vi "Simulador Circuito RLC- Gullit e Gabriela.vi"() -> ()   [LabVIEW 2020]
uses:
  <vilib>/Utility/file.llb/Read Delimited Spreadsheet (DBL).vi
  <vilib>/measure/NI_MABase.lvlib
panel:
  in  "i'(0)":dbl=1.0
  in  "i(0)":dbl
  in  "Vc'(0)":dbl=1.0
  in  "Vc(0)":dbl
  in  "C":dbl
  in  "L":dbl
  in  "R":dbl
  in  "Gerar ondas\nde saída":bool
  out "Tensão no Capacitor":cluster{dbl[], "Y":dbl[]}[](graph)
  out "Corrente":cluster{dbl[], "Y":dbl[]}[](graph)
  in  "Arquivo texto da onda":path
  out "Onda de entrada":cluster{dbl[], "Y":dbl[]}(graph)
  in  "Duty Cicle":dbl
  in  "Informação da amostragem":T1={"Taxa de amostragem"=1000.0, "N° de amostras"=100000.0} {"N° de amostras" format="%#.6g"; "Taxa de amostragem" format="%#.6g"}
  in  "Gerar onda \nde Entrada":bool
  in  "Tipo de Onda":u16(ring) items=["Senoidal", "Quadrada", "Onda qualquer", ""]
  in  "Amplitude":dbl
  in  "Frequência":dbl
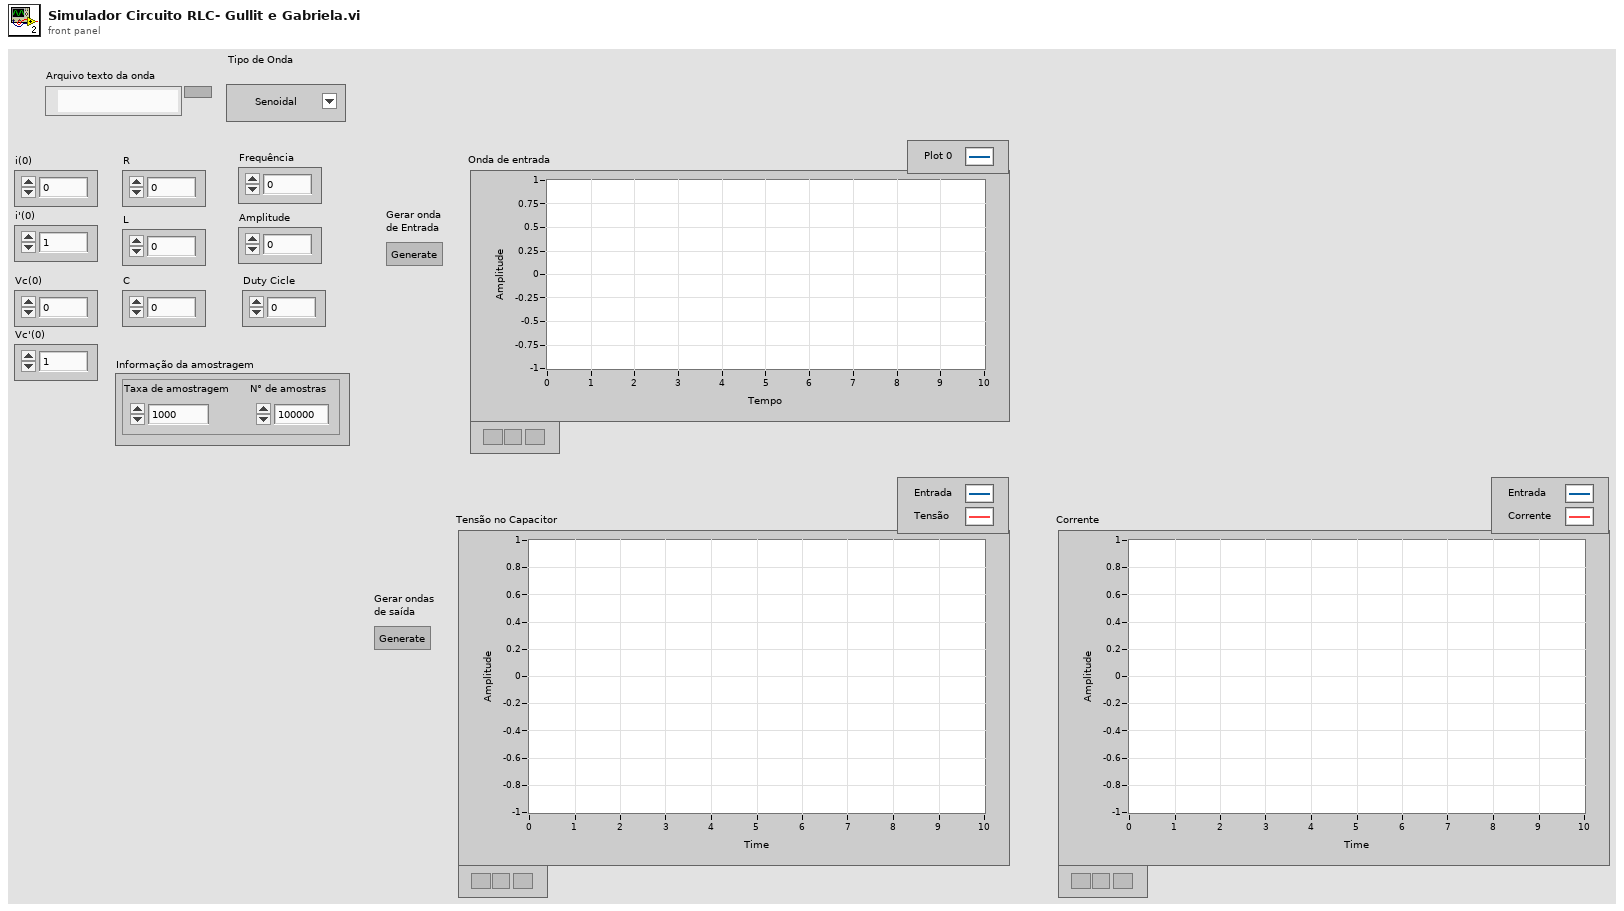
[diagram p1: front panel]
types:
  T1 = cluster{"Taxa de amostragem":dbl, "N° de amostras":dbl}
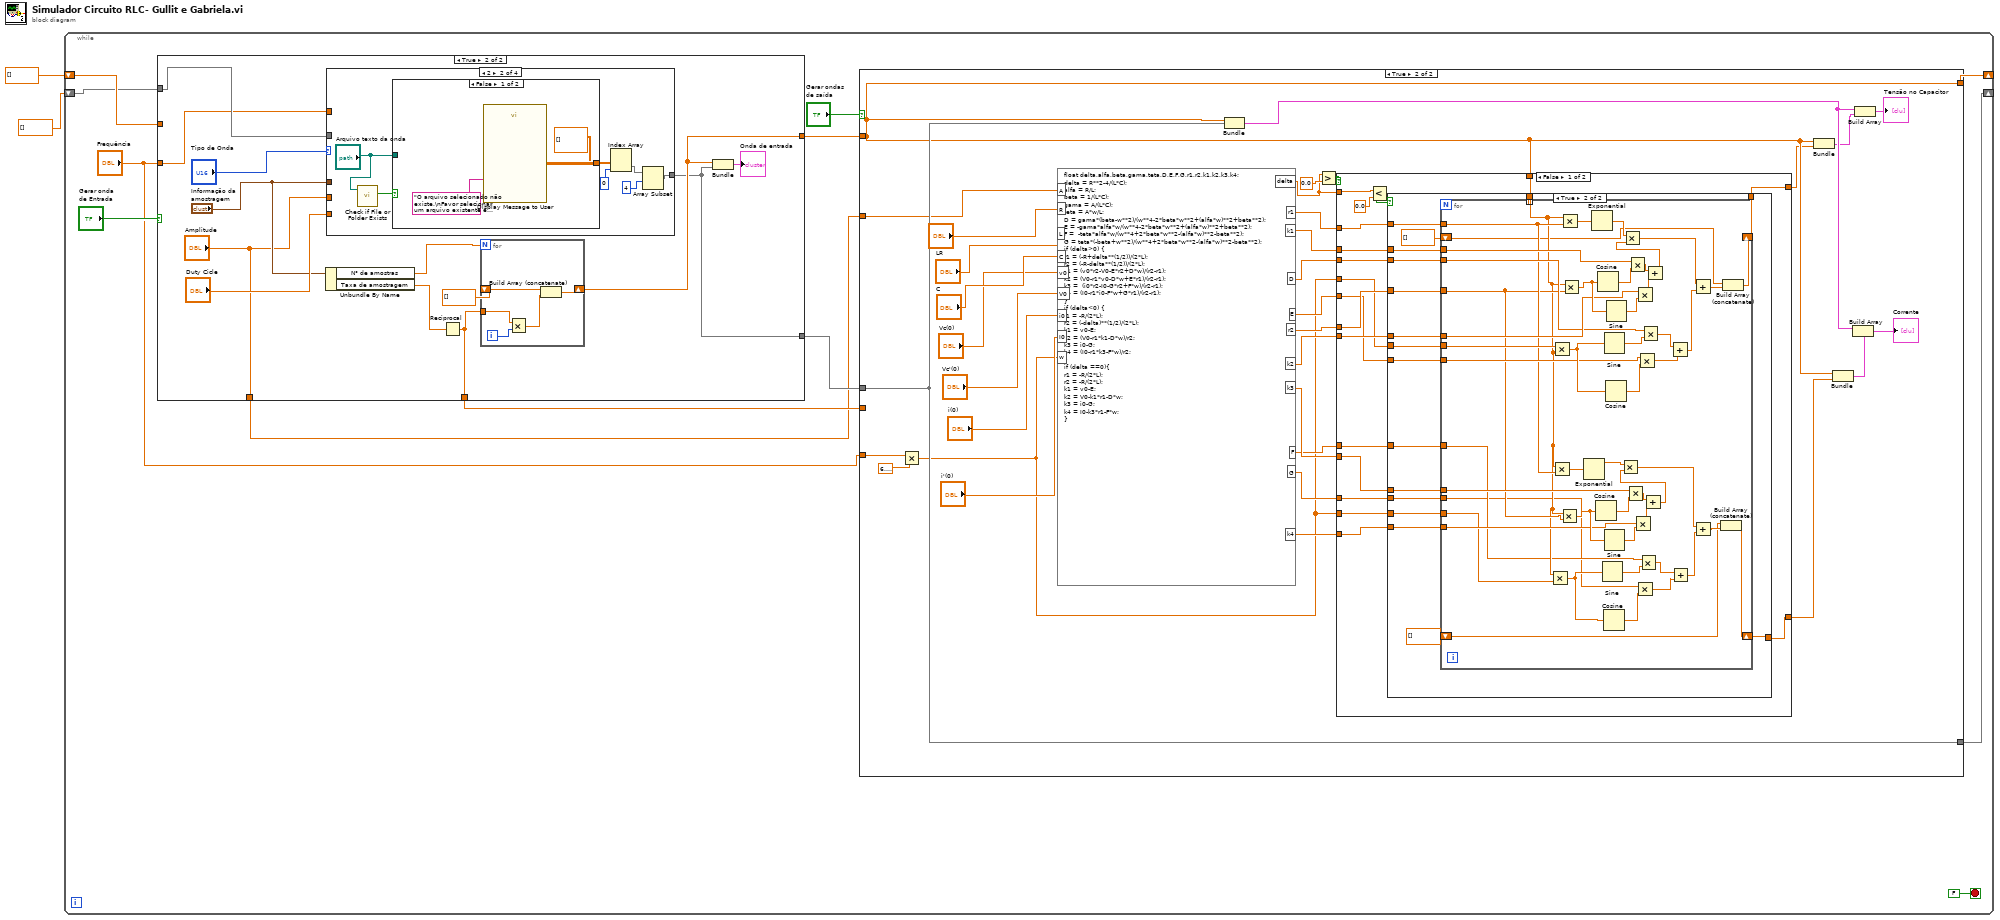
[diagram p0: block diagram]
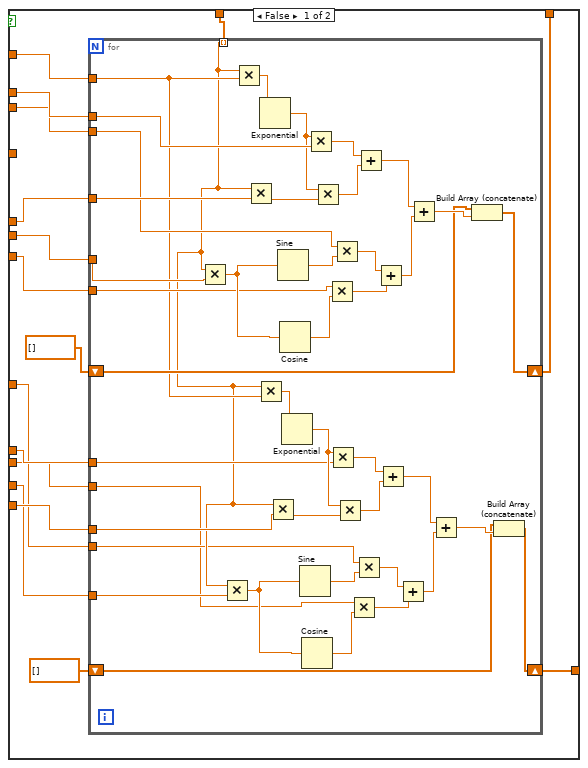
[diagram p3: hidden frame]
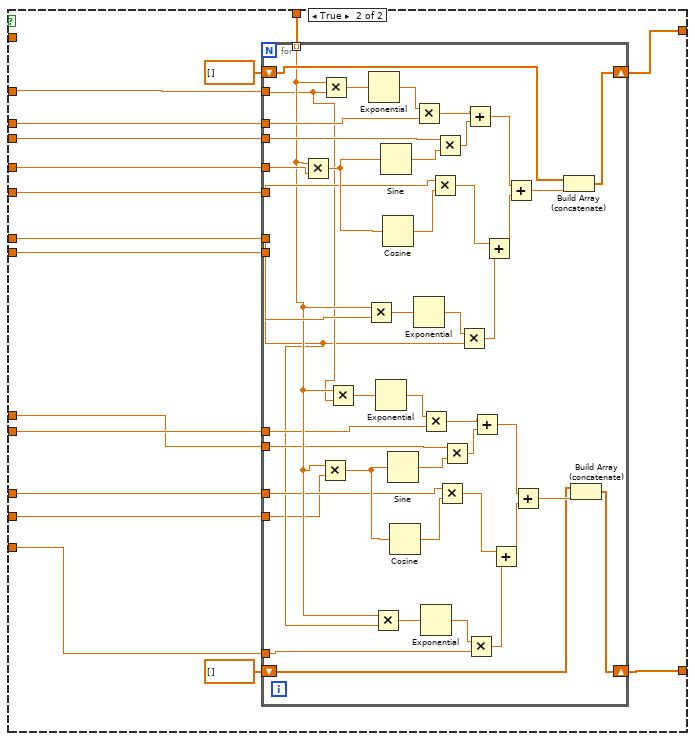
[diagram p4: hidden frame]
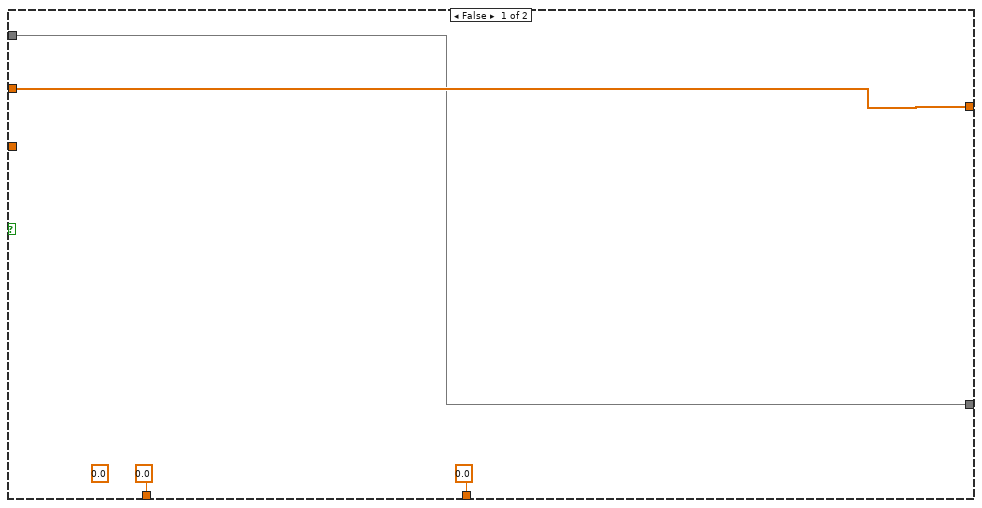
[diagram p5: hidden frame]
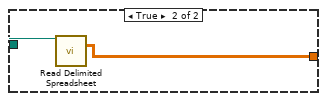
[diagram p7: hidden frame]
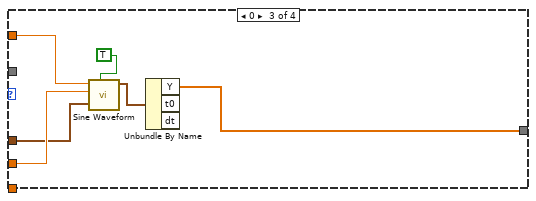
[diagram p8: hidden frame]
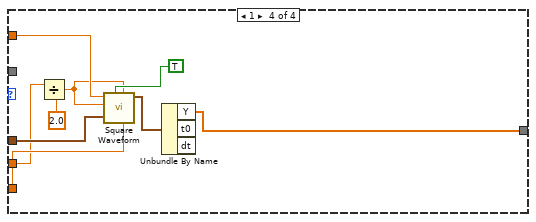
[diagram p9: hidden frame]
diagram:
  n1 = while {
    shift-right: [w10] -> _
    shift-left: dbl[] [] -> [w8]
    shift-right: [w9] -> _
    shift-left: dbl[] [] ("Y") -> [w7]
    stop <- FALSE stop-if-true
    n2 = case shown="True" "Gerar onda \nde Entrada" {
      tunnel: [w257 w264] -> w12
      tunnel: [w256 w263] -> w11
      tunnel: w8 -> [w257 _]
      tunnel: w7 -> [w256 w262]
      tunnel: [0.0 w260] -> w6
      tunnel: [0.0 ("Amplitude") "Amplitude"] -> w5
      tunnel: "Frequência" -> [_ w258]
      frame False {
        (unwired) 0.0 ("Frequência")
      }
      frame True {
        n3 = Unbundle By Name("Informação da amostragem") -> ("N° de amostras"=w266:dbl, "Taxa de amostragem"=w267:dbl)
        n4 = case shown="2" "Tipo de Onda" {
          tunnel: "Amplitude" -> [_ _ w292 w295]
          tunnel: w258 -> [_ _ w293 w302]
          tunnel: w262 -> [w276 _ _ _]
          tunnel: "Informação da amostragem" -> [_ _ w291 w301]
          tunnel: "Duty Cicle" -> [_ _ _ w300]
          tunnel: [w276 w279 w288 w297] -> w263
          frame Default {
          }
          frame 2 {
            n5 = call <vilib>:"Check if File or Folder Exists.vi"("path"="Arquivo texto da onda") -> ("file or folder exists?"=w277:bool)  [unwired: 8 in, 2 out]
            n6 = case shown="False" w277 {
              tunnel: "Arquivo texto da onda" -> [_ w287]
              tunnel: [dbl[][] [] ("all rows") w286] -> w281
              frame False {
                n7 = call "Display Message to User"("Message"="O arquivo selecionado não existe.\nFavor selecionar um arquivo existente e recomeçe a VI.") -> ()  [unwired: 9 in, 2 out]
              }
              frame True {
                n8 = call-poly <vilib>:"Read Delimited Spreadsheet.vi"("file path (dialog if empty)"=w287) -> ("all rows"=w286:dbl[][])  [unwired: 9 in, 5 out]
              }
            }
            n9 = Index Array(array=w281, index (col)=0 ("disabled index (col)")) -> (element=w282:dbl[])  [unwired: 1 in]
            n10 = Array Subset(array=w282, index=4) -> (w279:dbl[])  [unwired: 1 in]
          }
          frame 0 {
            n11 = call <vilib>:"Sine Waveform.vi"("sampling info"=w291, "reset signal"=TRUE, "amplitude"=w292, "frequency"=w293) -> ("signal out"=w289:waveform(dbl))  [unwired: 6 in, 1 out]
            n12 = Unbundle By Name(w289) -> ("Y"=w288:dbl[])  [unwired: 2 out]
          }
          frame 1 {
            n13 = Divide(x=w295, y=2.0) -> (x/y=w294:dbl)
            n14 = call <vilib>:"Square Waveform.vi"("duty cycle (%)"=w300, "offset"=w294, "sampling info"=w301, "reset signal"=TRUE, "amplitude"=w294, "frequency"=w302) -> ("signal out"=w298:waveform(dbl))  [unwired: 4 in, 1 out]
            n15 = Unbundle By Name(w298) -> ("Y"=w297:dbl[])  [unwired: 2 out]
          }
        }
        n16 = Reciprocal(x=w267) -> (1/x=w260:dbl)
        n17 = for {
          N: w266 -> [_]
          tunnel: w260 -> [w274]
          shift-right: [w272] -> w264
          shift-left: dbl[] [] -> [w271]
          i -> [w275]
          n18 = Multiply(x=w274, y=w275) -> (x*y=w273:dbl)
          n19 = Build Array (concatenate)(w271, w273) -> (w272:dbl[])
        }
        n20 = Bundle(w264, "Y"=w263) -> (→"Onda de entrada":cluster{dbl[], "Y":dbl[]})  [unwired: 1 in]
      }
    }
    n21 = case shown="True" "Gerar ondas\nde saída" {
      tunnel: w12 -> [w16 w37]
      tunnel: w11 -> [w15 w48]
      tunnel: [w16 w37] -> w10
      tunnel: [w15 w48] -> w9
      tunnel: w6 -> [_ _]
      tunnel: w5 -> [_ w42]
      tunnel: "Frequência" -> [_ w18]
      frame False {
      }
      frame True {
        n22 = Multiply(x=w18, y=6.283185307179586) -> (x*y=w17:dbl)
        n23 = formula code="float delta,alfa,beta,gama,teta,D,E,F,G,r1,r2,k1,k2,k3,k4;\ndelta = R**2-4/(L*C);\nalfa = R/L;\nbeta = 1/(L*C);\ngama = A/(L*C);\nteta = A*w/L;\nD = gama*(beta-w**2)/(w**4-2*beta*w**2+(alfa*w)**2+beta**2);\nE = -gama*alfa*w/(w**4-2*beta*w**2+(alfa*w)**2+beta**2);\nF =  -teta*alfa*w/(w**4+2*beta*w**2-(alfa*w)**2-beta**2);\nG = teta*(-beta+w**2)/(w**4+2*beta*w**2-(alfa*w)**2-beta**2);\nif (delta>0) {\nr1 = (-R+delta**(1/2))/(2*L);\nr2 = (-R-delta**(1/2))/(2*L);\nk1 = (v0*r2-V0-E*r2+D*w)/(r2-r1);\nk2 = (V0-r1*v0-D*w+E*r1)/(r2-r1);\nk3 =  (i0*r2-I0-G*r2+F*w)/(r2-r1);\nk4 = (I0-r1*i0-F*w+G*r1)/(r2-r1);\n}\nif (delta<0) {\nr1 = -R/(2*L);\nr2 = (-delta)**(1/2)/(2*L);\nk1 = v0-E;\nk2 = (V0-r1*k1-D*w)/r2;\nk3 = i0-G;\nk4 = (I0-r1*k3-F*w)/r2;\n}\nif (delta ==0){\nr1 = -R/(2*L);\nr2 = -R/(2*L);\nk1 = v0-E;\nk2 = V0-k1*r1-D*w;\nk3 = i0-G;\nk4 = I0-k3*r1-F*w;\n}"("C"="C", "L"="L", "R"="R", "A"=w42, "w"=w17, "v0"="Vc(0)", "V0"="Vc'(0)", "i0"="i(0)", "I0"="i'(0)") -> ("D"=w31:dbl, "E"=w32:dbl, "delta"=w24:dbl, "r1"=w36:dbl, "r2"=w34:dbl, "k1"=w35:dbl, "k2"=w33:dbl, "k3"=w28:dbl, "k4"=w25:dbl, "F"=w27:dbl, "G"=w26:dbl)
        n24 = Bundle(w37, "Y"=w48) -> (w49:cluster{dbl[], "Y":dbl[]})  [unwired: 1 in]
        n25 = Greater?(x=w24, y=0.0) -> (0:w40:bool)
        n26 = case shown="False" w40 {
          tunnel: w37 -> [w64 w208]
          tunnel: w36 -> [w63 w207]
          tunnel: w35 -> [w62 w206]
          tunnel: w34 -> [w61 w205]
          tunnel: w33 -> [w60 w204]
          tunnel: w17 -> [w59 w203]
          tunnel: w32 -> [w57 w202]
          tunnel: w31 -> [w58 w201]
          tunnel: w28 -> [w56 w199]
          tunnel: w27 -> [w53 w198]
          tunnel: w26 -> [w52 w197]
          tunnel: w25 -> [w54 w196]
          tunnel: w17 -> [w55 w194]
          tunnel: w24 -> [w66 _]
          tunnel: [w51 w193] -> w23
          tunnel: [w50 w192] -> w22
          frame False {
            n27 = Less?(x=w66, y=0.0) -> (x < y?=w67:bool)
            n28 = case shown="True" w67 {
              tunnel: w64 -> [w82 w139]
              tunnel: w63 -> [w81 w142]
              tunnel: w62 -> [w83 w141]
              tunnel: w61 -> [_ w140]
              tunnel: w60 -> [w80 w138]
              tunnel: w59 -> [w79 w137]
              tunnel: w58 -> [w78 w136]
              tunnel: w57 -> [w77 w135]
              tunnel: w56 -> [w75 w134]
              tunnel: w55 -> [w73 w133]
              tunnel: w54 -> [w74 w132]
              tunnel: w53 -> [w72 w131]
              tunnel: w52 -> [w71 w130]
              tunnel: [w69 w127] -> w51
              tunnel: [w68 w126] -> w50
              frame False {
                n29 = for {
                  tunnel: w83 -> [w125]
                  tunnel: w82 -> [w88] mode=indexing
                  tunnel: w81 -> [w92]
                  tunnel: w80 -> [w123]
                  tunnel: w79 -> [w113]
                  tunnel: w78 -> [w112]
                  tunnel: w77 -> [w111]
                  shift-right: [w107] -> w69
                  shift-left: dbl[] [] -> [w106]
                  tunnel: w75 -> [w91]
                  tunnel: w74 -> [w90]
                  tunnel: w73 -> [w89]
                  tunnel: w72 -> [w87]
                  tunnel: w71 -> [w86]
                  shift-right: [w85] -> w68
                  shift-left: dbl[] [] -> [w84]
                  n30 = Multiply(x=w88, y=w113) -> (x*y=w118:dbl)
                  n31 = Multiply(x=w88, y=w89) -> (x*y=w100:dbl)
                  n32 = Multiply(x=w88, y=w92) -> (x*y=w124:dbl)
                  n33 = Multiply(x=w88, y=w123) -> (x*y=w122:dbl)
                  n34 = Multiply(x=w88, y=w92) -> (x*y=w105:dbl)
                  n35 = Exponential(1:w124) -> (0:w121:dbl)
                  n36 = Multiply(x=w88, y=w90) -> (x*y=w104:dbl)
                  n37 = Sine(x=w118) -> (sin(x)=w116:dbl)
                  n38 = Cosine(x=w118) -> (cos(x)=w117:dbl)
                  n39 = Exponential(1:w105) -> (0:w103:dbl)
                  n40 = Sine(x=w100) -> (sin(x)=w98:dbl)
                  n41 = Cosine(x=w100) -> (cos(x)=w99:dbl)
                  n42 = Multiply(x=w121, y=w125) -> (x*y=w120:dbl)
                  n43 = Multiply(x=w121, y=w122) -> (x*y=w119:dbl)
                  n44 = Multiply(x=w111, y=w117) -> (x*y=w115:dbl)
                  n45 = Multiply(x=w103, y=w91) -> (x*y=w102:dbl)
                  n46 = Multiply(x=w112, y=w116) -> (x*y=w114:dbl)
                  n47 = Multiply(x=w103, y=w104) -> (x*y=w101:dbl)
                  n48 = Multiply(x=w86, y=w99) -> (x*y=w97:dbl)
                  n49 = Multiply(x=w87, y=w98) -> (x*y=w96:dbl)
                  n50 = Add(x=w120, y=w119) -> (x+y=w110:dbl)
                  n51 = Add(x=w114, y=w115) -> (x+y=w109:dbl)
                  n52 = Add(x=w102, y=w101) -> (x+y=w95:dbl)
                  n53 = Add(x=w96, y=w97) -> (x+y=w94:dbl)
                  n54 = Add(x=w110, y=w109) -> (x+y=w108:dbl)
                  n55 = Add(x=w95, y=w94) -> (x+y=w93:dbl)
                  n56 = Build Array (concatenate)(w106, w108) -> (w107:dbl[])
                  n57 = Build Array (concatenate)(w84, w93) -> (w85:dbl[])
                }
              }
              frame True {
                n58 = for {
                  tunnel: w142 -> [w172]
                  tunnel: w141 -> [w183]
                  tunnel: w140 -> [w159]
                  tunnel: w139 -> [w157] mode=indexing
                  tunnel: w138 -> [w179]
                  tunnel: w137 -> [w175]
                  tunnel: w136 -> [w174]
                  tunnel: w135 -> [w173]
                  tunnel: w134 -> [w162]
                  tunnel: w133 -> [w158]
                  tunnel: w132 -> [w161]
                  tunnel: w131 -> [w156]
                  tunnel: w130 -> [w155]
                  shift-right: [w146] -> w127
                  shift-left: dbl[] [] -> [w145]
                  shift-right: [w144] -> w126
                  shift-left: dbl[] [] -> [w143]
                  n59 = Multiply(x=w157, y=w158) -> (x*y=w171:dbl)
                  n60 = Multiply(x=w175, y=w157) -> (x*y=w189:dbl)
                  n61 = Multiply(x=w157, y=w172) -> (x*y=w184:dbl)
                  n62 = Multiply(x=w157, y=w159) -> (x*y=w167:dbl)
                  n63 = Multiply(x=w157, y=w172) -> (x*y=w191:dbl)
                  n64 = Multiply(x=w157, y=w159) -> (x*y=w181:dbl)
                  n65 = Exponential(1:w184) -> (0:w163:dbl)
                  n66 = Exponential(1:w191) -> (0:w190:dbl)
                  n67 = Cosine(x=w167) -> (cos(x)=w168:dbl)
                  n68 = Cosine(x=w181) -> (cos(x)=w182:dbl)
                  n69 = Sine(x=w171) -> (sin(x)=w169:dbl)
                  n70 = Cosine(x=w171) -> (cos(x)=w170:dbl)
                  n71 = Sine(x=w189) -> (sin(x)=w187:dbl)
                  n72 = Sine(x=w167) -> (sin(x)=w166:dbl)
                  n73 = Cosine(x=w189) -> (cos(x)=w188:dbl)
                  n74 = Sine(x=w181) -> (sin(x)=w180:dbl)
                  n75 = Multiply(x=w162, y=w168) -> (x*y=w165:dbl)
                  n76 = Multiply(x=w183, y=w182) -> (x*y=w178:dbl)
                  n77 = Multiply(x=w161, y=w166) -> (x*y=w164:dbl)
                  n78 = Multiply(x=w179, y=w180) -> (x*y=w177:dbl)
                  n79 = Multiply(x=w155, y=w170) -> (x*y=w153:dbl)
                  n80 = Multiply(x=w173, y=w188) -> (x*y=w149:dbl)
                  n81 = Multiply(x=w156, y=w169) -> (x*y=w154:dbl)
                  n82 = Multiply(x=w174, y=w187) -> (x*y=w148:dbl)
                  n83 = Add(x=w165, y=w164) -> (x+y=w160:dbl)
                  n84 = Multiply(x=w163, y=w160) -> (x*y=w151:dbl)
                  n85 = Add(x=w178, y=w177) -> (x+y=w176:dbl)
                  n86 = Multiply(x=w190, y=w176) -> (x*y=w147:dbl)
                  n87 = Add(x=w148, y=w149) -> (x+y=w186:dbl)
                  n88 = Add(x=w154, y=w153) -> (x+y=w152:dbl)
                  n89 = Add(x=w147, y=w186) -> (x+y=w185:dbl)
                  n90 = Add(x=w151, y=w152) -> (x+y=w150:dbl)
                  n91 = Build Array (concatenate)(w143, w150) -> (w144:dbl[])
                  n92 = Build Array (concatenate)(w145, w185) -> (w146:dbl[])
                }
              }
            }
          }
          frame True {
            n93 = for {
              tunnel: w208 -> [w218] mode=indexing
              tunnel: w207 -> [w217]
              tunnel: w206 -> [w253]
              tunnel: w205 -> [w248]
              tunnel: w204 -> [w212]
              tunnel: w203 -> [w247]
              tunnel: w202 -> [w244]
              tunnel: w201 -> [w242]
              shift-right: [w234] -> w193
              shift-left: dbl[] [] -> [w233]
              tunnel: w199 -> [w216]
              tunnel: w198 -> [w215]
              tunnel: w197 -> [w214]
              tunnel: w196 -> [w213]
              shift-right: [w211] -> w192
              shift-left: dbl[] [] -> [w210]
              tunnel: w194 -> [w209]
              n94 = Multiply(x=w218, y=w247) -> (x*y=w246:dbl)
              n95 = Multiply(x=w218, y=w209) -> (x*y=w228:dbl)
              n96 = Multiply(x=w218, y=w217) -> (x*y=w252:dbl)
              n97 = Multiply(x=w218, y=w217) -> (x*y=w232:dbl)
              n98 = Multiply(x=w218, y=w248) -> (x*y=w250:dbl)
              n99 = Exponential(1:w252) -> (0:w251:dbl)
              n100 = Multiply(x=w218, y=w212) -> (x*y=w230:dbl)
              n101 = Exponential(1:w232) -> (0:w231:dbl)
              n102 = Sine(x=w246) -> (sin(x)=w243:dbl)
              n103 = Cosine(x=w246) -> (cos(x)=w245:dbl)
              n104 = Sine(x=w228) -> (sin(x)=w226:dbl)
              n105 = Cosine(x=w228) -> (cos(x)=w227:dbl)
              n106 = Multiply(x=w251, y=w253) -> (x*y=w240:dbl)
              n107 = Exponential(1:w250) -> (0:w249:dbl)
              n108 = Multiply(x=w231, y=w216) -> (x*y=w224:dbl)
              n109 = Exponential(1:w230) -> (0:w229:dbl)
              n110 = Multiply(x=w244, y=w245) -> (x*y=w238:dbl)
              n111 = Multiply(x=w242, y=w243) -> (x*y=w241:dbl)
              n112 = Multiply(x=w214, y=w227) -> (x*y=w222:dbl)
              n113 = Multiply(x=w215, y=w226) -> (x*y=w225:dbl)
              n114 = Multiply(x=w249, y=w212) -> (x*y=w239:dbl)
              n115 = Add(x=w240, y=w241) -> (x+y=w236:dbl)
              n116 = Multiply(x=w229, y=w213) -> (x*y=w223:dbl)
              n117 = Add(x=w224, y=w225) -> (x+y=w220:dbl)
              n118 = Add(x=w238, y=w239) -> (x+y=w237:dbl)
              n119 = Add(x=w222, y=w223) -> (x+y=w221:dbl)
              n120 = Add(x=w236, y=w237) -> (x+y=w235:dbl)
              n121 = Add(x=w220, y=w221) -> (x+y=w219:dbl)
              n122 = Build Array (concatenate)(w233, w235) -> (w234:dbl[])
              n123 = Build Array (concatenate)(w210, w219) -> (w211:dbl[])
            }
          }
        }
        n124 = Bundle(w37, w23) -> (w20:cluster{dbl[], dbl[]})  [unwired: 1 in]
        n125 = Bundle(w37, w22) -> (w21:cluster{dbl[], dbl[]})  [unwired: 1 in]
        n126 = Build Array(w49, w21) -> (→"Corrente":cluster{dbl[], "Y":dbl[]}[])
        n127 = Build Array(w49, w20) -> (→"Tensão no Capacitor":cluster{dbl[], "Y":dbl[]}[])
      }
    }
  }
